vi "main.vi"() -> ()   [LabVIEW 2020]
uses:
  <vilib>/DAQmx/write.llb/DAQmx Write (Analog 1D DBL NChan 1Samp).vi
  <vilib>/DAQmx/create/channels.llb/DAQmx Create Channel (AO-Voltage-Basic).vi
  <vilib>/DAQmx/miscellaneous.llb/DAQmx Fill In Error Info.vi
panel:
  out "Emitting:":bool=TRUE
  in  "Shutter 2":bool
  in  "Power (%)":dbl(slide)=100.0 scale=0.0..100.0
  out "Emitting:":bool=TRUE
  in  "stop":bool
  in  "Shutter":bool
  in  "Power (%)":dbl(slide)=100.0 scale=0.0..100.0
  # "Analog control AOMs Salix"
  # "515 nm"
  # "561 nm"
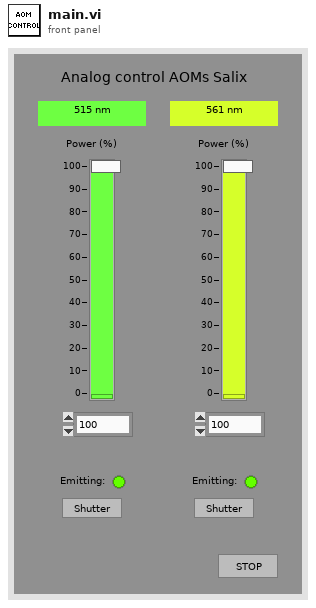
[diagram p1: front panel]
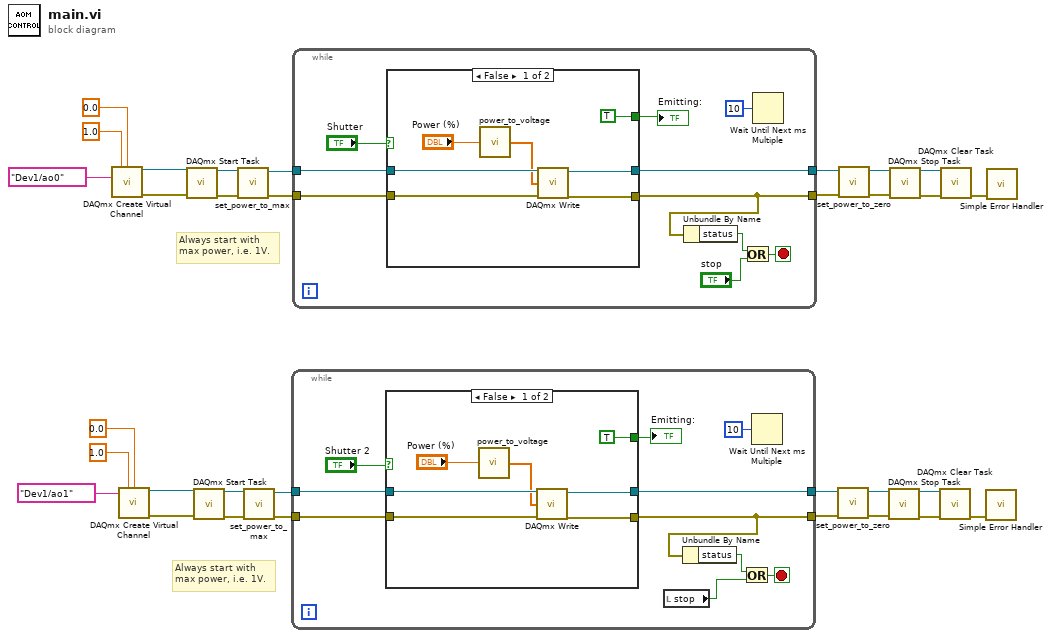
[diagram p0: block diagram]
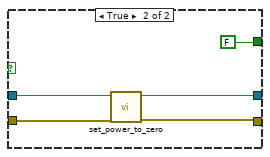
[diagram p2: hidden frame]
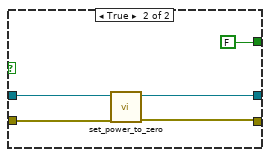
[diagram p3: hidden frame]
diagram:
  # "Always start with\nmax power, i.e. 1V."
  # "Always start with\nmax power, i.e. 1V."
  n1 = call-poly <vilib>:"DAQmx Create Virtual Channel.vi"("maximum value"=1.0, "minimum value"=0.0, "physical channels"=tag "Dev1/ao0") -> ("task out"=w29:refnum<k21>, "error out"=w28:errorcluster)  [unwired: 11 in]
  n2 = call-poly <vilib>:"DAQmx Create Virtual Channel.vi"("maximum value"=1.0, "minimum value"=0.0, "physical channels"=tag "Dev1/ao1") -> ("task out"=w18:refnum<k21>, "error out"=w17:errorcluster)  [unwired: 11 in]
  n3 = call <vilib>:"DAQmx Start Task.vi"("task/channels in"=w29, "error in"=w28) -> ("task out"=w4:refnum<k21>, "error out"=w3:errorcluster)  [unwired: 12 in]
  n4 = call <vilib>:"DAQmx Start Task.vi"("task/channels in"=w18, "error in"=w17) -> ("task out"=w8:refnum<k21>, "error out"=w7:errorcluster)  [unwired: 12 in]
  n5 = call "set_power_to_max.vi"("error in"=w3, "task/channels in"=w4) -> ("error out"=w1:errorcluster, "task out"=w2:refnum<k21>)  [unwired: 8 in]
  n6 = call "set_power_to_max.vi"("error in"=w7, "task/channels in"=w8) -> ("error out"=w5:errorcluster, "task out"=w6:refnum<k21>)  [unwired: 8 in]
  n7 = while {
    tunnel: w6 -> [w41]
    tunnel: w5 -> [w40]
    tunnel: [w38] -> w11
    tunnel: [w37] -> w12
    stop <- w42 stop-if-true
    n8 = case shown="False" "Shutter 2" {
      tunnel: w41 -> [w49 w53]
      tunnel: w40 -> [w48 w51]
      tunnel: [w47 w50] -> w38
      tunnel: [w46 w52] -> w37
      tunnel: [TRUE ("Boolean") FALSE ("Boolean")] -> w34
      frame False {
        n9 = call "power_to_voltage.vi"("Power (%)"="Power (%)") -> ("Voltage"=w45:dbl[])
        n10 = call-poly <vilib>:"DAQmx Write.vi"("task/channels in"=w49, "data"=w45, "error in"=w48) -> ("task out"=w46:refnum<k21>, "error out"=w47:errorcluster)  [unwired: 10 in, 1 out]
      }
      frame True {
        n11 = call "set_power_to_zero.vi"("error in"=w51, "task/channels in"=w53) -> ("error out"=w50:errorcluster, "task out"=w52:refnum<k21>)  [unwired: 8 in]
      }
    }
    "Emitting:" <- w34
    n12 = local read "stop"() -> (w33:bool)
    n13 = Unbundle By Name(w38) -> ("status"=w39:bool)
    n14 = Or(x=w39, y=w33) -> (x .or. y?=w42:bool)
    n15 = Wait Until Next ms Multiple(millisecond multiple=u32 10) -> ()  [unwired: 1 out]
  }
  n16 = while {
    tunnel: w2 -> [w63]
    tunnel: w1 -> [w62]
    tunnel: [w60] -> w22
    tunnel: [w59] -> w23
    stop <- w64 stop-if-true
    n17 = case shown="False" "Shutter" {
      tunnel: w63 -> [w71 w75]
      tunnel: w62 -> [w70 w73]
      tunnel: [w69 w72] -> w60
      tunnel: [w68 w74] -> w59
      tunnel: [TRUE ("Boolean") FALSE ("Boolean")] -> w56
      frame False {
        n18 = call "power_to_voltage.vi"("Power (%)"="Power (%)") -> ("Voltage"=w67:dbl[])
        n19 = call-poly <vilib>:"DAQmx Write.vi"("task/channels in"=w71, "data"=w67, "error in"=w70) -> ("task out"=w68:refnum<k21>, "error out"=w69:errorcluster)  [unwired: 10 in, 1 out]
      }
      frame True {
        n20 = call "set_power_to_zero.vi"("error in"=w73, "task/channels in"=w75) -> ("error out"=w72:errorcluster, "task out"=w74:refnum<k21>)  [unwired: 8 in]
      }
    }
    "Emitting:" <- w56
    n21 = Unbundle By Name(w60) -> ("status"=w61:bool)
    n22 = Or(x=w61, y="stop") -> (x .or. y?=w64:bool)
    n23 = Wait Until Next ms Multiple(millisecond multiple=u32 10) -> ()  [unwired: 1 out]
  }
  n24 = call "set_power_to_zero.vi"("error in"=w11, "task/channels in"=w12) -> ("error out"=w13:errorcluster, "task out"=w14:refnum<k21>)  [unwired: 8 in]
  n25 = call "set_power_to_zero.vi"("error in"=w22, "task/channels in"=w23) -> ("error out"=w24:errorcluster, "task out"=w25:refnum<k21>)  [unwired: 8 in]
  n26 = call <vilib>:"DAQmx Stop Task.vi"("task/channels in"=w14, "error in"=w13) -> ("task out"=w21:refnum<k21>, "error out"=w20:errorcluster)  [unwired: 12 in]
  n27 = call <vilib>:"DAQmx Stop Task.vi"("task/channels in"=w25, "error in"=w24) -> ("task out"=w32:refnum<k21>, "error out"=w31:errorcluster)  [unwired: 12 in]
  n28 = call <vilib>:"DAQmx Clear Task.vi"("task in"=w21, "error in"=w20) -> ("error out"=w19:errorcluster)  [unwired: 13 in]
  n29 = call <vilib>:"DAQmx Clear Task.vi"("task in"=w32, "error in"=w31) -> ("error out"=w30:errorcluster)  [unwired: 13 in]
  n30 = call <vilib>:"Simple Error Handler.vi"("error in (no error)"=w19) -> ()  [unwired: 4 in, 5 out]
  n31 = call <vilib>:"Simple Error Handler.vi"("error in (no error)"=w30) -> ()  [unwired: 4 in, 5 out]
